vi "Build High Priority Execute.vi"(6 "Group":i32, 7 "Virtual Memory Unit in":refnum<class "Virtual Memory Unit.lvclass">, 8 "error in (no error)":errorcluster, 10 "Starting Address":u16 format="%04x", 11 "Major Frame in":refnum<class "Major Frame.lvclass">) -> (0 "error out":errorcluster, 2 "Next Available Address":u16 format="%04x", 3 "Major Frame out":refnum<class "Major Frame.lvclass">, 5 "Virtual Memory Unit out":refnum<class "Virtual Memory Unit.lvclass">)   [LabVIEW 2020, in "BCI-1553 API.lvlib" / "Major Frame.lvclass"]
doc: "Builds the high priority message execution code."
uses:
  Major Frame.lvclass
  Dependencies/Virtual Memory Unit/Virtual Memory Unit.lvclass
  TypeDefs/BC Op Codes - Verbose.ctl
  TypeDefs/BC Condition Codes.ctl
  Major Frame.lvclass/Major Frame.ctl
  BCI-1553 API.lvlib
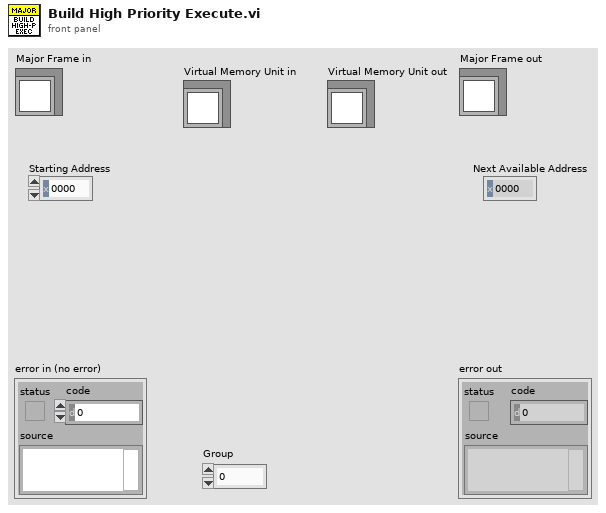
[diagram p1: front panel]
types:
  T1 = typedef "BCI-1553 API.lvlib/BC Condition Codes.ctl" = enum16{"GP0 == 1 || LT", "GP1 == 1 || NE", "GP2 == 1", "GP3 == 1", "GP4 == 1", "GP5 == 1", "GP6 == 1", "GP7 == 1", "NORESP", "FMTERR", "GOODBLOCK", "MSKSTATSET", "BADMSG", "1RETRY", "2RETRY", "ALWAYS"}
  T2 = typedef "BCI-1553 API.lvlib/BC Op Codes - Verbose.ctl" = enum16{"EXECUTE MSG", "EXECUTE MSG GO", "JUMP", "CALL SUBROUTINE", "RETURN", "INTERRUPT REQUEST", "HALT", "DELAY", "WAIT FRAME TIMER = 0", "COMPARE FRAME TIMER", "COMPARE MSG TIMER", "LOAD TIME TAG CTR", "LOAD TIME TAG CTR HI", "LOAD FRAME TIMER", "START FRAME TIMER", "PUSH TIME TAG COUNT", "PUSH TIME TAG COUNT HI", "PUSH TIME TAG COUNT BOTH", "PUSH BLOCK STATUS WORD", "PUSH CURRENT VALUE", "PUSH INDIRECT", "WAIT EXT TRIGGER", "EXECUTE AND FLIP", "EXECUTE, FLIP, GO", "WRITE VALUE TO WMI", "WRITE VALUE TO MEM", "DECREMENT RAM, SKIP", "FLAG"}
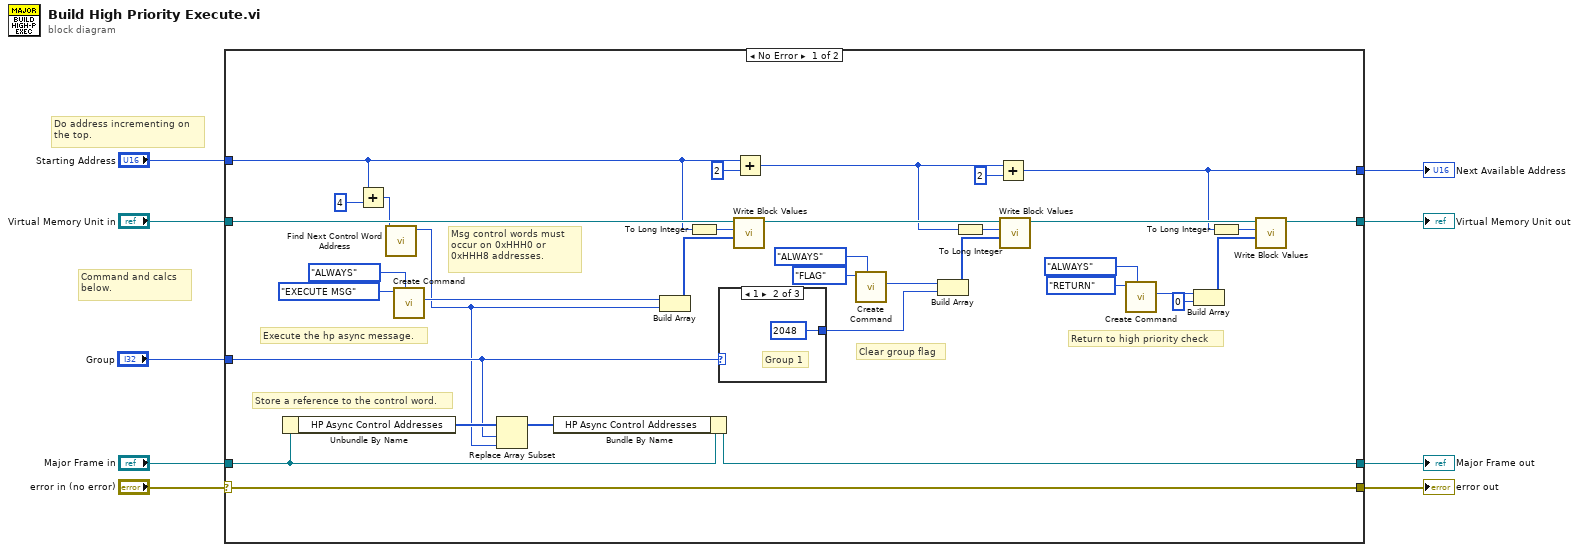
[diagram p0: block diagram]
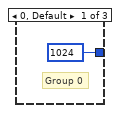
[diagram p2: hidden frame]
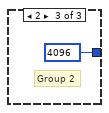
[diagram p3: hidden frame]
diagram:
  # "Command and calcs\nbelow."
  # "Do address incrementing on\nthe top."
  n1 = case shown="No Error" "error in (no error)" {
    selector: "error in (no error)" -> [w21 w49]
    tunnel: [w21 w49] -> w6
    tunnel: [w16 w48] -> w5
    tunnel: "Major Frame in" -> [w17 w48]
    tunnel: "Virtual Memory Unit in" -> [w42 _]
    tunnel: [w32 _] -> w3
    tunnel: "Starting Address" -> [w12 _]
    tunnel: [w10 _] -> w4
    tunnel: "Group" -> [w19 _]
    frame No Error {
      # "Store a reference to the control word."
      # "Msg control words must\noccur on 0xHHH0 or \n0xHHH8 addresses."
      # "Clear group flag"
      # "Return to high priority check"
      # "Execute the hp async message."
      n2 = Unbundle By Name(w17) -> ("HP Async Control Addresses"=w20:u16[])
      n3 = Add(x=w12, y=u16 4) -> (x+y=w11:u16)
      n4 = call "Find Next Control Word Address.vi"("Starting Address"=w11) -> ("0xHHHX Address"=w14:u16)  [unwired: 10 in]
      n5 = call "Create Command.vi"("Condition"=BC_Condition_Codes."ALWAYS", "Op Code"=BC_Op_Codes_-_Verbose."EXECUTE MSG") -> ("Instruction"=w18:u16)  [unwired: 8 in, 1 out]
      n6 = Replace Array Subset(array=w20, new element=w14, index=w19) -> (w15:u16[])
      n7 = Bundle By Name(cluster=w17, "HP Async Control Addresses"=w15) -> (w16:refnum<class "Major Frame.lvclass">)
      n8 = Build Array(w18, w14) -> (w41:u16[])
      n9 = To Long Integer(number=w12) -> (32bit integer=w40:i32)
      n10 = case shown="1" w19 {
        tunnel: [u16 1024 ("element") u16 2048 ("element") u16 4096 ("element")] -> w22
        frame 0, Default {
          # "Group 0"
        }
        frame 1 {
          # "Group 1"
        }
        frame 2 {
          # "Group 2"
        }
      }
      n11 = call "Write Block Values.vi"("Write Block"=w41, "Start Index"=w40, "Virtual Memory Unit in"=w42) -> ("Virtual Memory Unit out"=w26:refnum<class "Virtual Memory Unit.lvclass">)  [unwired: 7 in, 1 out]
      n12 = Add(x=w12, y=u16 2) -> (x+y=w23:u16)
      n13 = call "Create Command.vi"("Condition"=BC_Condition_Codes."ALWAYS", "Op Code"=BC_Op_Codes_-_Verbose."FLAG") -> ("Instruction"=w29:u16)  [unwired: 8 in, 1 out]
      n14 = Build Array(w29, w22) -> (w30:u16[])
      n15 = To Long Integer(number=w23) -> (32bit integer=w31:i32)
      n16 = Add(x=w23, y=u16 2) -> (x+y=w10:u16)
      n17 = call "Write Block Values.vi"("Write Block"=w30, "Start Index"=w31, "Virtual Memory Unit in"=w26) -> ("Virtual Memory Unit out"=w25:refnum<class "Virtual Memory Unit.lvclass">)  [unwired: 7 in, 1 out]
      n18 = call "Create Command.vi"("Condition"=BC_Condition_Codes."ALWAYS", "Op Code"=BC_Op_Codes_-_Verbose."RETURN") -> ("Instruction"=w34:u16)  [unwired: 8 in, 1 out]
      n19 = Build Array(w34, u16 0 ("element")) -> (w36:u16[])
      n20 = To Long Integer(number=w10) -> (32bit integer=w35:i32)
      n21 = call "Write Block Values.vi"("Write Block"=w36, "Start Index"=w35, "Virtual Memory Unit in"=w25) -> ("Virtual Memory Unit out"=w32:refnum<class "Virtual Memory Unit.lvclass">)  [unwired: 7 in, 1 out]
    }
    frame Error {
    }
  }
  "error out" <- w6
  "Major Frame out" <- w5
  "Virtual Memory Unit out" <- w3
  "Next Available Address" <- w4
